vi "DistanceToTarget.vi"() -> ()   [LabVIEW 2019]
panel:
  in  "Distance":dbl
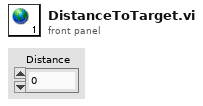
[diagram p1: front panel]
diagram:
